vi "f2.vi"(2 "Numeric 2":dbl, 3 "Numeric":dbl) -> (0 "Numeric 4":dbl, 1 "Numeric 3":dbl)   [LabVIEW 2020]
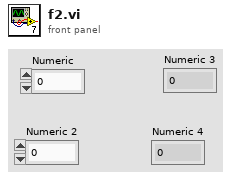
[diagram p1: front panel]
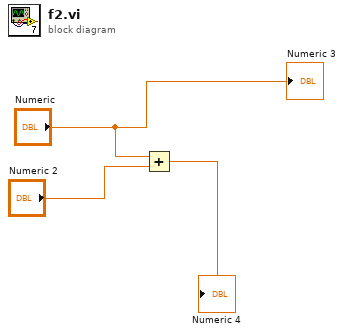
[diagram p0: block diagram]
diagram:
  n1 = Add(x="Numeric", y="Numeric 2") -> (x+y=→"Numeric 4":dbl)
  "Numeric 3" <- "Numeric"
